vi "FGV_GUI_reference.vi"(7 "FGV states":T1, 8 "error in (no error)":errorcluster, 11 "Button refs In":T2) -> (0 "error out":errorcluster, 3 "Button refs Out":T2)   [LabVIEW 2021]
uses:
  CTLs/ButtonRefs.ctl
  CTLs/playback status.ctl
  FGVstates.ctl
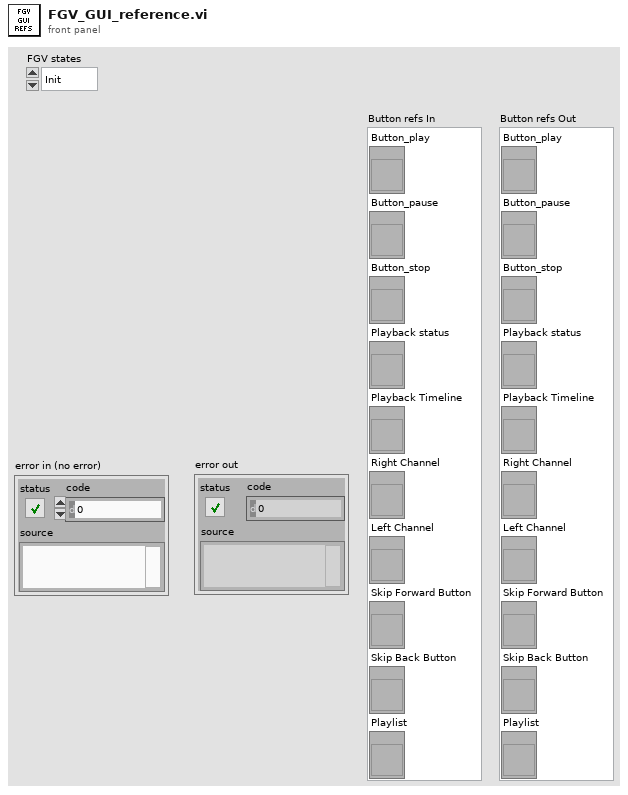
[diagram p1: front panel]
types:
  T1 = typedef "FGVstates.ctl" = enum16{"Init", "Set", "Get", "De-Init"}
  T2 = typedef "ButtonRefs.ctl" = cluster{"Button_play":refnum<vi>, "Button_pause":refnum<vi>, "Button_stop":refnum<vi>, "Playback status":refnum<vi>, "Playback Timeline":refnum<vi>, "Right Channel":refnum<vi>, "Left Channel":refnum<vi>, "Skip Forward Button":refnum<vi>, "Skip Back Button":refnum<vi>, "Playlist":refnum<vi>}
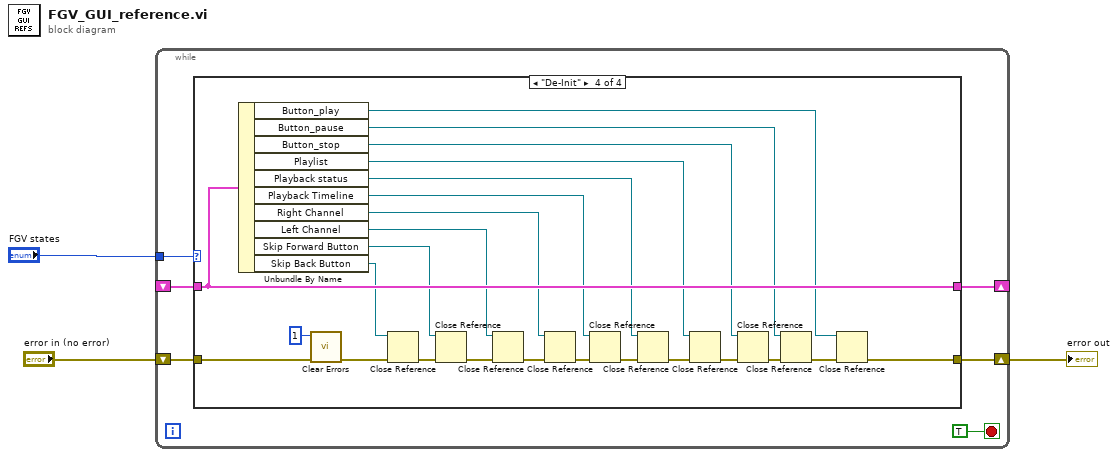
[diagram p0: block diagram]
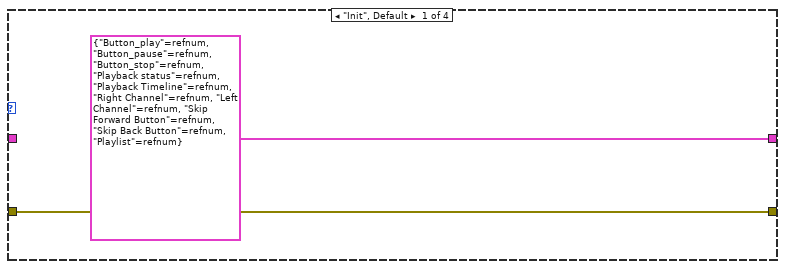
[diagram p2: hidden frame]
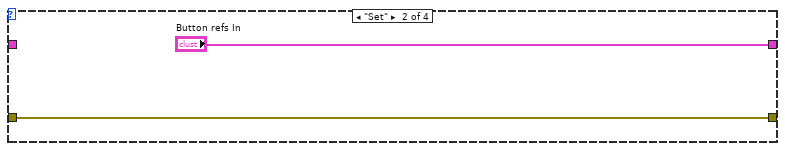
[diagram p3: hidden frame]
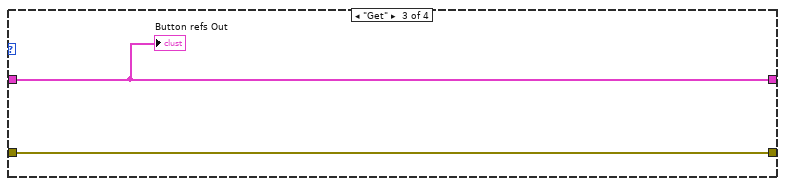
[diagram p4: hidden frame]
diagram:
  n1 = while {
    tunnel: "FGV states" -> [w9]
    shift-right: [w7] -> w1
    shift-left: "error in (no error)" -> [w8]
    shift-right: [w5] -> _
    shift-left: _ -> [w4]
    stop <- TRUE stop-if-true
    n2 = case shown="\"De-Init\"" w9 {
      tunnel: w8 -> [w11 w13 w15 w18]
      tunnel: [w11 w13 w15 w16] -> w7
      tunnel: [T2 {"Button_play"=refnum, "Button_pause"=refnum, "Button_stop"=refnum, "Playback status"=refnum, "Playback Timeline"=refnum, "Right Channel"=refnum, "Left Channel"=refnum, "Skip Forward Button"=refnum, "Skip Back Button"=refnum, "Playlist"=refnum} ("Button refs") "Button refs In" w14 w39] -> w5
      tunnel: w4 -> [_ _ w14 w39]
      frame "Init", Default {
      }
      frame "Set" {
      }
      frame "Get" {
        "Button refs Out" <- w14
      }
      frame "De-Init" {
        n3 = Unbundle By Name(w39) -> ("Button_play"=w20:refnum<vi>, "Button_pause"=w21:refnum<vi>, "Button_stop"=w22:refnum<vi>, "Playlist"=w23:refnum<vi>, "Playback status"=w29:refnum<vi>, "Playback Timeline"=w30:refnum<vi>, "Right Channel"=w31:refnum<vi>, "Left Channel"=w32:refnum<vi>, "Skip Forward Button"=w33:refnum<vi>, "Skip Back Button"=w34:refnum<vi>)
        n4 = call <vilib>:"Clear Errors.vi"("error in (no error)"=w18, "specific error code to clear (0: all)"=1) -> ("error out"=w19:errorcluster)  [unwired: 4 in, 1 out]
        n5 = Close Reference(reference=w34, error in (no error)=w19) -> (error out=w35:errorcluster)
        n6 = Close Reference(reference=w33, error in (no error)=w35) -> (error out=w36:errorcluster)
        n7 = Close Reference(reference=w32, error in (no error)=w36) -> (error out=w37:errorcluster)
        n8 = Close Reference(reference=w31, error in (no error)=w37) -> (error out=w38:errorcluster)
        n9 = Close Reference(reference=w30, error in (no error)=w38) -> (error out=w28:errorcluster)
        n10 = Close Reference(reference=w29, error in (no error)=w28) -> (error out=w24:errorcluster)
        n11 = Close Reference(reference=w23, error in (no error)=w24) -> (error out=w25:errorcluster)
        n12 = Close Reference(reference=w22, error in (no error)=w25) -> (error out=w26:errorcluster)
        n13 = Close Reference(reference=w21, error in (no error)=w26) -> (error out=w27:errorcluster)
        n14 = Close Reference(reference=w20, error in (no error)=w27) -> (error out=w16:errorcluster)
      }
    }
  }
  "error out" <- w1
